vi "Read Settings.vi"(8 "error in (no error)":errorcluster, 11 "ESP301 in":refnum<class "ESP301.lvclass">) -> (0 "error out":errorcluster, 2 "Settings":T1={"devport"="COM3", "Position"={"Axis 1"={"Value"=0.0024, "Min"=0.0, "Max"=2.9, "StepSize"=0.001, "Tolerance"=0.0001, "ValueActual"=0.0}, "Axis 2"={"Value"=0.0, "Min"=0.0, "Max"=2.9, "StepSize"=0.001, "Tolerance"=0.0001, "ValueActual"=0.0}, "Axis 3"={"Value"=0.0, "Min"=0.0, "Max"=2.9, "StepSize"=0.001, "Tolerance"=0.0001, "ValueActual"=0.0}}, "Power"={"Axis 1"=enum."on", "Axis 2"=enum."on", "Axis 3"=enum."on"}, "Status"={"Axis 1"=enum."Not referenced", "Axis 2"=enum."Not referenced", "Axis 3"=enum."Not referenced"}, "Backlash"={"Axis 1"={"Value"=0.0, "Min"=0.0, "Max"=4.0, "StepSize"=0.1, "Tolerance"=0.01, "ValueActual"=0.0}, "Axis 2"={"Value"=0.0, "Min"=0.0, "Max"=4.0, "StepSize"=0.1, "Tolerance"=0.01, "ValueActual"=0.0}, "Axis 3"={"Value"=0.0, "Min"=0.0, "Max"=4.0, "StepSize"=0.1, "Tolerance"=0.01, "ValueActual"=0.0}}, "Home"={"Axis 1"={"Value"=0.0, "Min"=0.0, "Max"=6.0, "StepSize"=0.001, "Tolerance"=0.0001, "ValueActual"=0.0}, "Axis 2"={"Value"=0.0, "Min"=0.0, "Max"=6.0, "StepSize"=0.001, "Tolerance"=0.0001, "ValueActual"=0.0}, "Axis 3"={"Value"=0.0, "Min"=0.0, "Max"=6.0, "StepSize"=0.001, "Tolerance"=0.0001, "ValueActual"=0.0}}, "MoveToHardLimit"={"Axis 1"=enum."neg", "Axis 2"=enum."neg", "Axis 3"=enum."neg"}, "relativeMove"={"Axis 1neg"=enum."off", "Axis 2neg"=enum."off", "Axis 3neg"=enum."off", "Axis 1pos"=enum."off", "Axis 2pos"=enum."off", "Axis 3pos"=enum."off"}, "stepsize"={"Value"=0.01, "Min"=0.0, "Max"=1.0, "StepSize"=0.01, "Tolerance"=0.0001, "ValueActual"=0.0}, "automotoroff"=enum."off", "ResetBeforeMove"=enum."off", "Enable"={"Axis 1"=enum."off", "Axis 2"=enum."off", "Axis 3"=enum."on"}, "InitWithDBValues"=enum."off"}, 3 "ESP301 out":refnum<class "ESP301.lvclass">)   [LabVIEW 2020, in "ESP301.lvclass"]
uses:
  ESP301.lvclass
  SettingsTypdef.ctl
  OnOffTypeDef.ctl
  status_TypDef.ctl
  Hardware limit.ctl
  ESP301.lvclass/ESP301.ctl
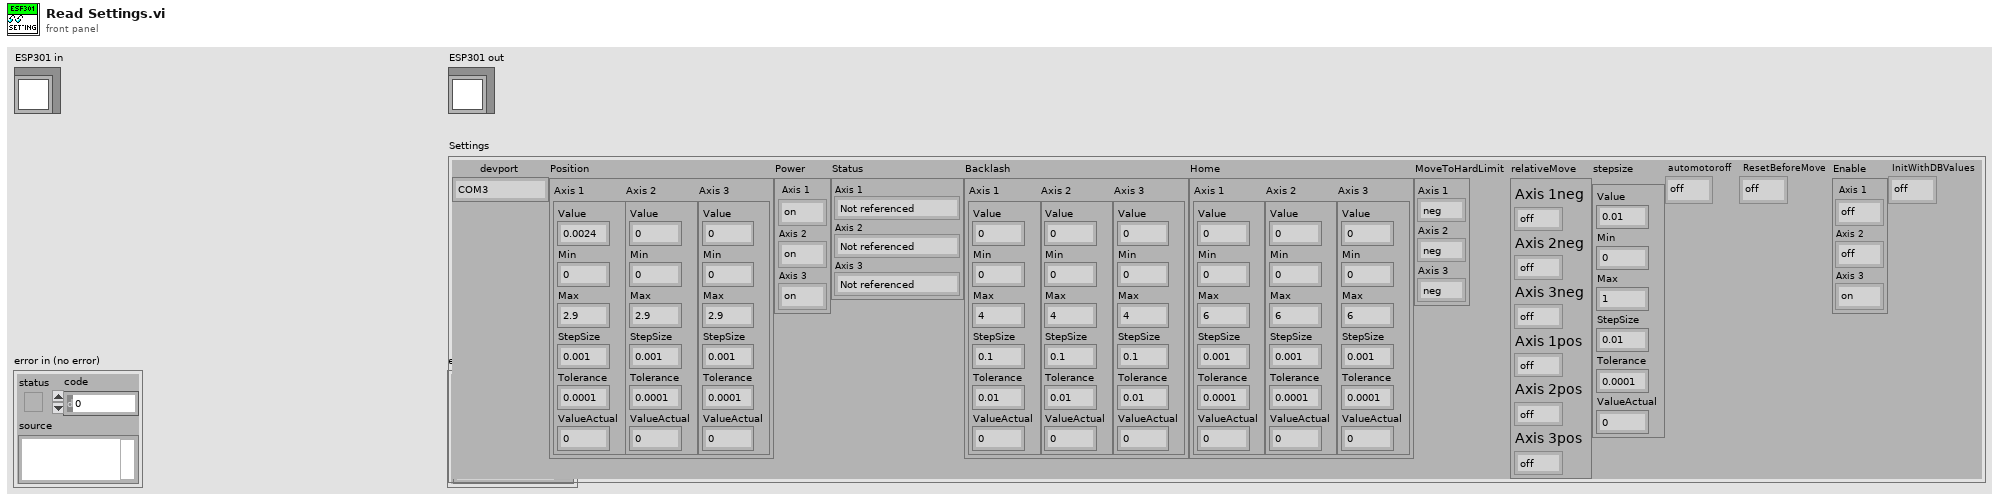
[diagram p1: front panel]
types:
  T1 = typedef "ESP301.lvclass/SettingsTypdef.ctl" = cluster{"devport":string, "Position":cluster{"Axis 1":cluster{"Value":dbl, "Min":dbl, "Max":dbl, "StepSize":dbl, "Tolerance":dbl, "ValueActual":dbl}, "Axis 2":cluster{"Value":dbl, "Min":dbl, "Max":dbl, "StepSize":dbl, "Tolerance":dbl, "ValueActual":dbl}, "Axis 3":cluster{"Value":dbl, "Min":dbl, "Max":dbl, "StepSize":dbl, "Tolerance":dbl, "ValueActual":dbl}}, "Power":cluster{"Axis 1":T2, "Axis 2":T2, "Axis 3":T2}, "Status":cluster{"Axis 1":T3, "Axis 2":T3, "Axis 3":T3}, "Backlash":cluster{"Axis 1":cluster{"Value":dbl, "Min":dbl, "Max":dbl, "StepSize":dbl, "Tolerance":dbl, "ValueActual":dbl}, "Axis 2":cluster{"Value":dbl, "Min":dbl, "Max":dbl, "StepSize":dbl, "Tolerance":dbl, "ValueActual":dbl}, "Axis 3":cluster{"Value":dbl, "Min":dbl, "Max":dbl, "StepSize":dbl, "Tolerance":dbl, "ValueActual":dbl}}, "Home":cluster{"Axis 1":cluster{"Value":dbl, "Min":dbl, "Max":dbl, "StepSize":dbl, "Tolerance":dbl, "ValueActual":dbl}, "Axis 2":cluster{"Value":dbl, "Min":dbl, "Max":dbl, "StepSize":dbl, "Tolerance":dbl, "ValueActual":dbl}, "Axis 3":cluster{"Value":dbl, "Min":dbl, "Max":dbl, "StepSize":dbl, "Tolerance":dbl, "ValueActual":dbl}}, "MoveToHardLimit":cluster{"Axis 1":T4, "Axis 2":T4, "Axis 3":T4}, "relativeMove":cluster{"Axis 1neg":T2, "Axis 2neg":T2, "Axis 3neg":T2, "Axis 1pos":T2, "Axis 2pos":T2, "Axis 3pos":T2}, "stepsize":cluster{"Value":dbl, "Min":dbl, "Max":dbl, "StepSize":dbl, "Tolerance":dbl, "ValueActual":dbl}, "automotoroff":T2, "ResetBeforeMove":T2, "Enable":cluster{"Axis 1":T2, "Axis 2":T2, "Axis 3":T2}, "InitWithDBValues":T2}
  T2 = typedef "OnOffTypeDef.ctl" = enum16{"off", "on"}
  T3 = typedef "status_TypDef.ctl" = enum16{"Not referenced", "Homing", "Moving", "Ready"}
  T4 = typedef "Hardware limit.ctl" = enum16{"pos", "neg"}
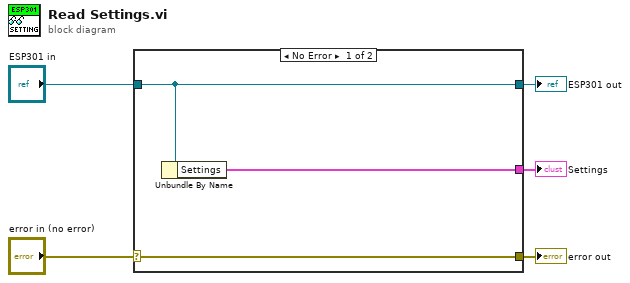
[diagram p0: block diagram]
diagram:
  n1 = case shown="No Error" "error in (no error)" {
    selector: "error in (no error)" -> [w8 w9]
    tunnel: [w8 w9] -> w4
    tunnel: [w7 w10] -> w2
    tunnel: "ESP301 in" -> [w7 w10]
    tunnel: [w6 _] -> w1
    frame No Error {
      n2 = Unbundle By Name(w7) -> ("Settings"=w6:T1)
    }
    frame Error {
    }
  }
  "error out" <- w4
  "ESP301 out" <- w2
  "Settings" <- w1
